vi "CHD_DRIVE_Get_KINEMATIC.vi"() -> (1 "out DIFF_DRIVE_KINEMATICS":T1 {"TrackWidth_Meters" format="%20.4f"})   [LabVIEW 2019]
uses:
  <vilib>/Rock Robotics/WPI/ThirdParty/JAS_Junk/TrajLib/TypeDef/DIFF_DRIVE_KINEMATICS.ctl
  CHD_DRIVE_GLOBALS.vi
  <vilib>/Rock Robotics/WPI/ThirdParty/JAS_Junk/TrajLib/Trajectory_Library.lvlib
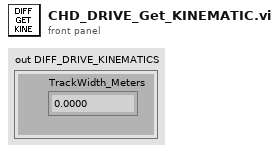
[diagram p1: front panel]
types:
  T1 = typedef "Trajectory_Library.lvlib/DIFF_DRIVE_KINEMATICS.ctl" = cluster{"TrackWidth_Meters":dbl}
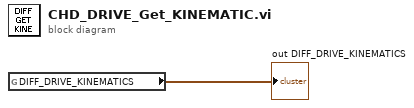
[diagram p0: block diagram]
diagram:
  n1 = global read "CHD_DRIVE_GLOBALS.vi" "DIFF_DRIVE_KINEMATICS"() -> (→"out DIFF_DRIVE_KINEMATICS":T1)
